vi "Next Action Core.vi"(11 "Actions":string) -> (1 "Arguments":string, 2 "Next Action":string, 3 "Remaining Actions":string)   [LabVIEW 2020, in "Action Stack.lvlib"]
doc: "Parses the Action list and returns the next action with the associated arguments.\n\nThis provides the functionality to the JKI Statemachine \"Parse State Queue\" vi, but without the error input.\n\n<B>Action Syntax:</B>\nAction >> Argument\nAction separator: Line feed\nTo add a comment use \"//\" or \"#\" and all text to the right will be ignored\n\n<B>Example:</B>\n//Initial Actions\nUI:Initialize // This initializes the UI\nData:Initialize\nUpdate // initial update"
uses:
  <vilib>/JDP Science/JDP Science Common Utilities/Action Stack/Action Stack.lvlib
  <vilib>/JDP Science/JDP Science Common Utilities/JDP Utility.lvlib
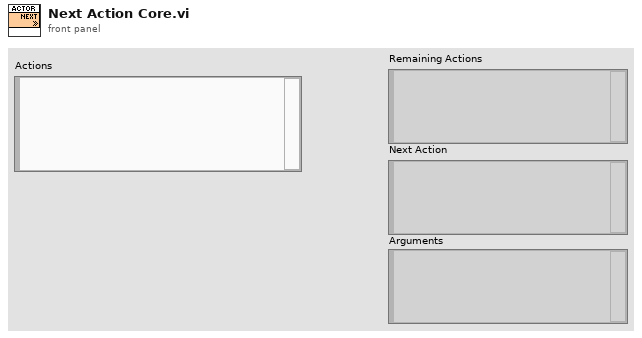
[diagram p1: front panel]
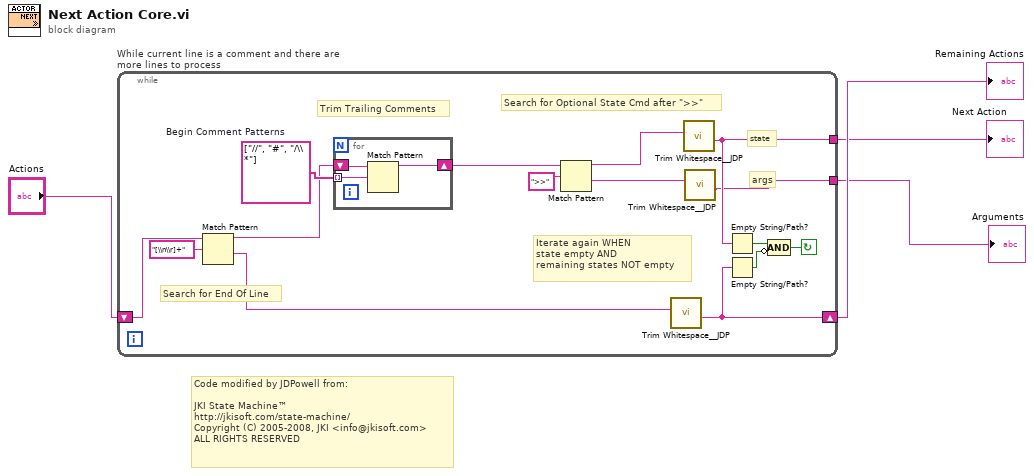
[diagram p0: block diagram]
diagram:
  # "Code modified by JDPowell from:\n\nJKI State Machine™\nhttp://jkisoft.com/state-machine/\nCopyright (C) 2005-2008, JKI <info@jkisoft.com>\nALL RIGHTS RESERVED"
  n1 = while "While current line is a comment and there are more lines to process" {
    tunnel: [w9] -> w3
    tunnel: [w7] -> w2
    shift-right: [w5] -> w4
    shift-left: "Actions" -> [w13]
    stop <- w15 continue-if-true
    w19 = string[] ["//", "#", "/\\*"]  # Begin Comment Patterns
    # "Search for End Of Line"
    # "Iterate again WHEN\nstate empty AND\nremaining states NOT empty"
    # "args"
    # "state"
    # "Search for Optional State Cmd after \">>\""
    # "Trim Trailing Comments"
    n2 = Match Pattern(string=w13, regular expression="[\\n\\r]+") -> (before substring=w12:string, after substring=w6:string)  [unwired: 1 in, 2 out]
    n3 = for {
      tunnel: w19 -> [w21] mode=indexing
      shift-right: [w20] -> w11
      shift-left: w12 -> [w22]
      n4 = Match Pattern(string=w22, regular expression=w21) -> (before substring=w20:string)  [unwired: 1 in, 3 out]
    }
    n5 = Match Pattern(string=w11, regular expression=">>") -> (before substring=w10:string, after substring=w8:string)  [unwired: 1 in, 2 out]
    n6 = call <vilib>:"Trim Whitespace__JDP.vi"("String in"=w6) -> ("String out"=w5:string)  [unwired: 6 in]
    n7 = call <vilib>:"Trim Whitespace__JDP.vi"("String in"=w10) -> ("String out"=w9:string)  [unwired: 6 in]
    n8 = call <vilib>:"Trim Whitespace__JDP.vi"("String in"=w8) -> ("String out"=w7:string)  [unwired: 6 in]
    n9 = Empty String/Path?(string/path=w9) -> (empty?=w17:bool)
    n10 = Empty String/Path?(string/path=w5) -> (empty?=w16:bool)
    n11 = Compound Arithmetic op=AND(w17, invert w16) -> (w15:bool)
  }
  "Remaining Actions" <- w4
  "Next Action" <- w3
  "Arguments" <- w2
